vi "Get Properties.vi"(8 "error in (no error)":errorcluster, 11 "Acrobat Template in":refnum<class "Application.lvclass">) -> (0 "error out":errorcluster, 2 "Class Properties":T1 {"Mode" items=["Operator"=0, "Engineering"=1, "Verification"=6]}, 3 "Acrobat Template out":refnum<class "Application.lvclass">)   [LabVIEW 2017, in "Application.lvlib" / "Application.lvclass"]
uses:
  Application.lvclass
  Properties/Class Properties -- Cluster.ctl
  Golden Board/Class/Golden Board.lvclass
  Test Recipe/Class/Test Recipe.lvclass
  Station Config/Class/Station Config.lvclass
  <vilib>/TSS/ACRObat Test Framework/Classes/Variable Engine/Class/Variable Engine.lvclass
  Properties/UUT Reference -- Cluster.ctl
  typedefs/Test Info -- Cluster.ctl
  Instruments/Instrument/Class/Instrument.lvclass
  typedefs/Op Mode -- Enum.ctl
  Properties/Test Result -- Cluster.ctl
  Application.lvclass/Application.ctl
  Properties/App Properties.lvclass
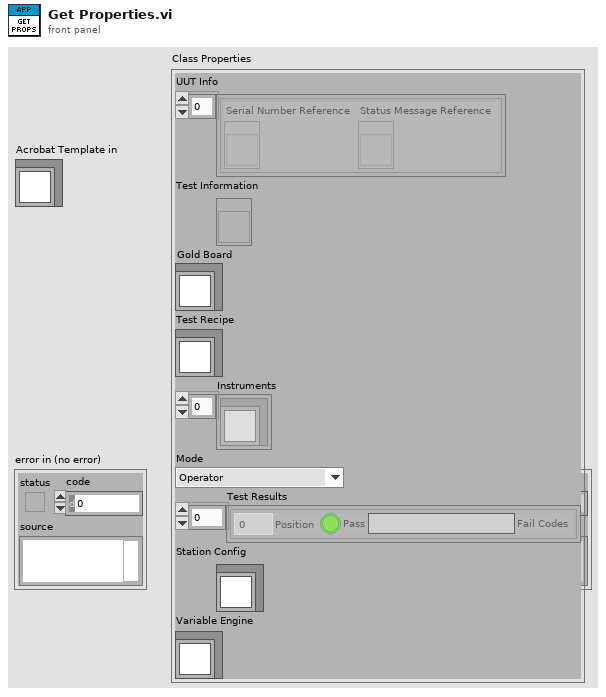
[diagram p1: front panel]
types:
  T1 = typedef "Application.lvlib/App Properties.lvclass/Class Properties -- Cluster.ctl" = cluster{"UUT Info":T2[], "Test Information":refnum<vi>, "Gold Board":refnum<class "Golden Board.lvclass">, "Test Recipe":refnum<class "Test Recipe.lvclass">, "Instruments":refnum<class "Instrument.lvclass">[], "Mode":T3, "Test Results":T4[], "Station Config":refnum<class "Station Config.lvclass">, "Variable Engine":refnum<class "Variable Engine.lvclass">}
  T2 = typedef "Application.lvlib/App Properties.lvclass/UUT Reference -- Cluster.ctl" = cluster{"Serial Number Reference":refnum<vi>, "Status Message Reference":refnum<vi>}
  T3 = typedef "Application.lvlib/Application.lvclass/Op Mode -- Enum.ctl" = u16
  T4 = typedef "Application.lvlib/App Properties.lvclass/Test Result -- Cluster.ctl" = cluster{"Position":i32, "Pass":bool, "Fail Codes":string}
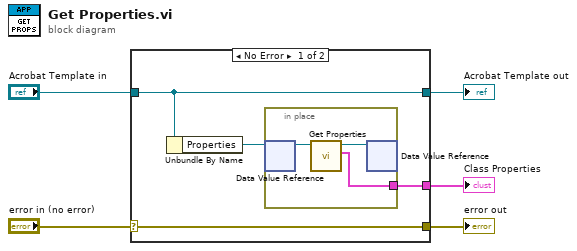
[diagram p0: block diagram]
diagram:
  n1 = case shown="No Error" "error in (no error)" {
    selector: "error in (no error)" -> [w9 w14]
    tunnel: [w9 w14] -> w4
    tunnel: [w8 w13] -> w2
    tunnel: "Acrobat Template in" -> [w8 w13]
    tunnel: [w6 _] -> w1
    frame No Error {
      n2 = Unbundle By Name(w8) -> ("Properties"=w7:refnum<data-value>)
      n3 = in-place {
        in-place-border: [w10] -> w6
        n4 = in-place-dvr #1(w7) -> (w12:refnum<class "App Properties.lvclass">)  [unwired: 1 out]
        n5 = call-dynamic "Get Properties.vi"("App Properties in"=w12) -> ("Class Properties"=w10:T1, "App Properties out"=w11:refnum<class "App Properties.lvclass">)  [unwired: 8 in, 1 out]
        n6 = in-place-dvr #1(w11) -> ()  [unwired: 2 out]
      }
    }
    frame Error {
    }
  }
  "error out" <- w4
  "Acrobat Template out" <- w2
  "Class Properties" <- w1
